vi "init_dataframe.vi"(10 "data":string, 11 "type":u8) -> (3 "DataFrame.lvclass":refnum<class "DataFrame.lvclass">)   [LabVIEW 2017, in "DataFrame.lvclass"]
uses:
  DataFrame.lvclass
  DataFrame.lvclass/DataFrame.ctl
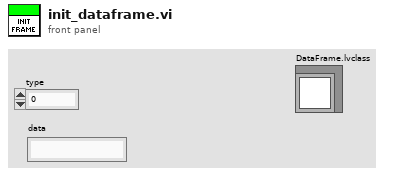
[diagram p1: front panel]
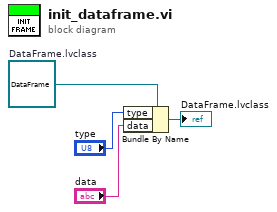
[diagram p0: block diagram]
diagram:
  w4 = refnum<class "DataFrame.lvclass"> refnum  # DataFrame.lvclass
  n1 = Bundle By Name(cluster=w4, "type"="type", "data"="data") -> (→"DataFrame.lvclass":refnum<class "DataFrame.lvclass">)
